vi "SetLaunchInputs.vi"(5 "enableDefaultFile":bool, 7 "defaultFileAppender":T3={"common"={"id"="", "threshold"=enum."INFO", "filter"={"mode"=enum."Mirror", "levelMin"=enum."INFO", "levelMax"=enum."INFO", "tagPrefix"=""}, "queueBound"=0, "dropPolicy"=enum."DropOldest", "useUTC"=FALSE}, "file"={"rootFolder"=path "", "maxFileSize"=0, "maxFileCount"=0, "baseName"="", "extension"="", "delimiter"="", "calendarFolderTree"=FALSE}}, 8 "error in (no error)":errorcluster, 10 "ManagerLaunchInputs":T1={"initialGlobalThreshold"=enum."INFO", "hostApplicationPath"=path "", "configFilePath"=path "", "snapshotNotifier"=refnum, "stoppedNotifier"=refnum}, 11 "LogManager in":refnum<class "LogManager.lvclass">) -> (0 "error out":errorcluster, 3 "LogManager out":refnum<class "LogManager.lvclass">)   [LabVIEW 2026, in "Lumberjack.lvlib" / "LogManager.lvclass"]
doc: "Stash the LogManager's launch inputs (initial global threshold, default file appender config, config file path, host application path, and the shared Snapshot notifier) into private data before launch. Called by Initialize prior to Launch Root Actor; Actor Core reads these on entry to resolve config and post the initial snapshot."
uses:
  LogManager.lvclass
  TypeDefs/Severity.ctl
  TypeDefs/FileAppenderConfig.ctl
  TypeDefs/AppenderConfig.ctl
  TypeDefs/Filter.ctl
  TypeDefs/FilterMode.ctl
  TypeDefs/DropPolicy.ctl
  TypeDefs/FileConfig.ctl
  TypeDefs/Snapshot.ctl
  <vilib>/ActorFramework/Message Enqueuer/Message Enqueuer.lvclass
  LogManager.lvclass/LogManager.ctl
  Lumberjack.lvlib
  TypeDefs/ManagerLaunchInputs.ctl
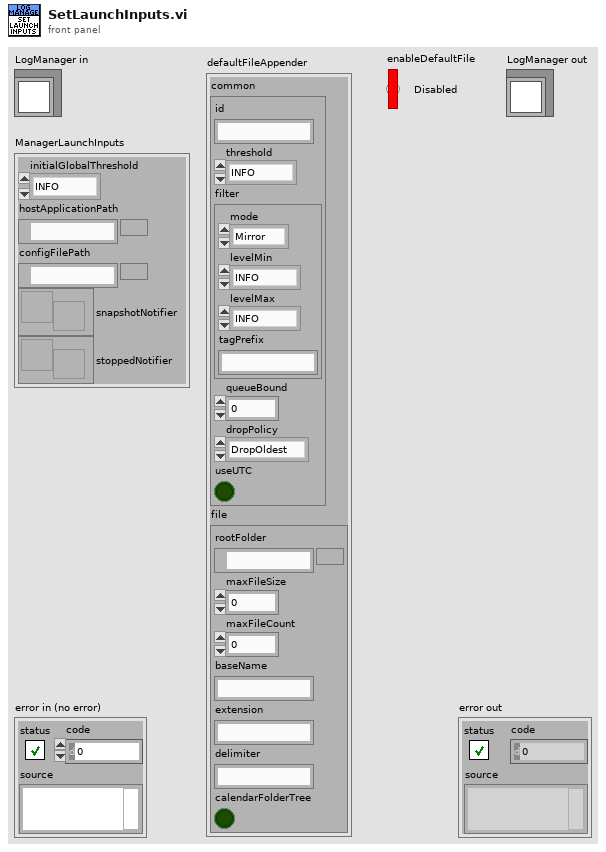
[diagram p1: front panel]
types:
  T1 = typedef "Lumberjack.lvlib/ManagerLaunchInputs.ctl" = cluster{"initialGlobalThreshold":T2, "hostApplicationPath":path, "configFilePath":path, "snapshotNotifier":refnum<notifier>, "stoppedNotifier":refnum<notifier>}
  T2 = typedef "Lumberjack.lvlib/Severity.ctl" = enum16{"OFF", "FATAL", "ERROR", "WARN", "INFO", "DEBUG", "TRACE", "ALL"}
  T3 = typedef "Lumberjack.lvlib/FileAppenderConfig.ctl" = cluster{"common":T4, "file":T8}
  T4 = typedef "Lumberjack.lvlib/AppenderConfig.ctl" = cluster{"id":string, "threshold":T2, "filter":T5, "queueBound":i32, "dropPolicy":T7, "useUTC":bool}
  T5 = typedef "Lumberjack.lvlib/Filter.ctl" = cluster{"mode":T6, "levelMin":T2, "levelMax":T2, "tagPrefix":string}
  T6 = typedef "Lumberjack.lvlib/FilterMode.ctl" = enum16{"Mirror", "Routed"}
  T7 = typedef "Lumberjack.lvlib/DropPolicy.ctl" = enum16{"DropOldest", "DropNewest", "LevelAware"}
  T8 = typedef "Lumberjack.lvlib/FileConfig.ctl" = cluster{"rootFolder":path, "maxFileSize":i64, "maxFileCount":i32, "baseName":string, "extension":string, "delimiter":string, "calendarFolderTree":bool}
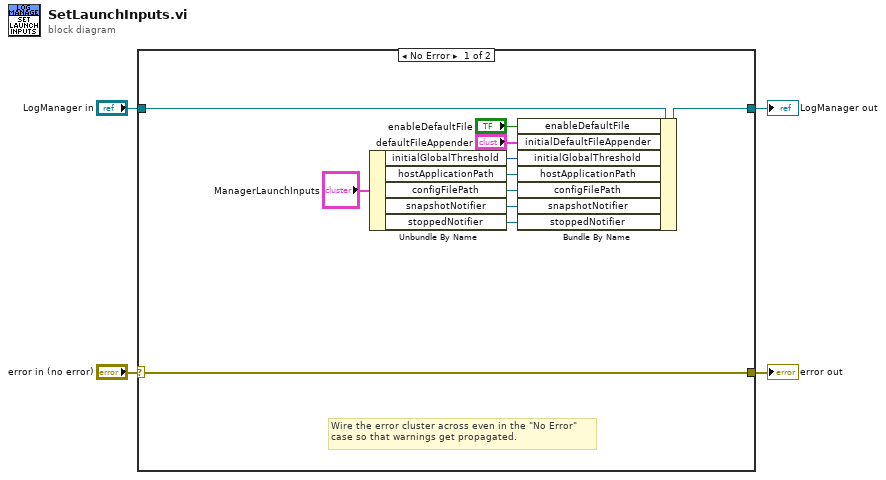
[diagram p0: block diagram]
diagram:
  n1 = case shown="No Error" "error in (no error)" {
    selector: "error in (no error)" -> [w15 w17]
    tunnel: [w15 w17] -> w3
    tunnel: [w14 w16] -> w1
    tunnel: "LogManager in" -> [w13 w16]
    frame No Error {
      # "Wire the error cluster across even in the \"No Error\"\ncase so that warnings get propagated."
      n2 = Unbundle By Name("ManagerLaunchInputs") -> ("initialGlobalThreshold"=w9:T2, "hostApplicationPath"=w8:path, "configFilePath"=w7:path, "snapshotNotifier"=w6:refnum<notifier>, "stoppedNotifier"=w5:refnum<notifier>)
      n3 = Bundle By Name(cluster=w13, "enableDefaultFile"="enableDefaultFile", "initialDefaultFileAppender"="defaultFileAppender", "initialGlobalThreshold"=w9, "hostApplicationPath"=w8, "configFilePath"=w7, "snapshotNotifier"=w6, "stoppedNotifier"=w5) -> (w14:refnum<class "LogManager.lvclass">)
    }
    frame Error {
    }
  }
  "error out" <- w3
  "LogManager out" <- w1
